vi "Periodic Tasks.vi"(8 "error in":errorcluster) -> ()   [LabVIEW 2016]
doc: "This VI runs in parallel to other tasks. It can contain as many user-defined periodic loops as you need. These can carry out PID or other sorts of timed response."
uses:
  <vilib>/Rock Robotics/WPI/Utilities/WPI_GetSetVariantRefNum.vi
  <vilib>/Rock Robotics/Network Tables/NT Write Number.vi
  2_11_17/Systems/Global 1.vi
  <vilib>/Analysis/NI_AALBase.lvlib
  <vilib>/Instr/_visa.llb/VISA Configure Serial Port (Instr).vi
  <vilib>/Analysis/3filter.llb/IIR Filter (DBL).vi
panel:
  out "PSI":dbl
  in  "off set":dbl=55.0 format="%#_13g"
  out "read buffer":string="B:3,X:197.00,Y:124.00"
  in  "Search_Params":string[](array[string])=["B", "X", "Y", "W1", "H1", "W2", "H2"]
  out "Last Complete Message":string="B:2,X:197.00,Y:124.00,W1:9,H1:24,W2:9,H2:23"
  out "length":i32=43
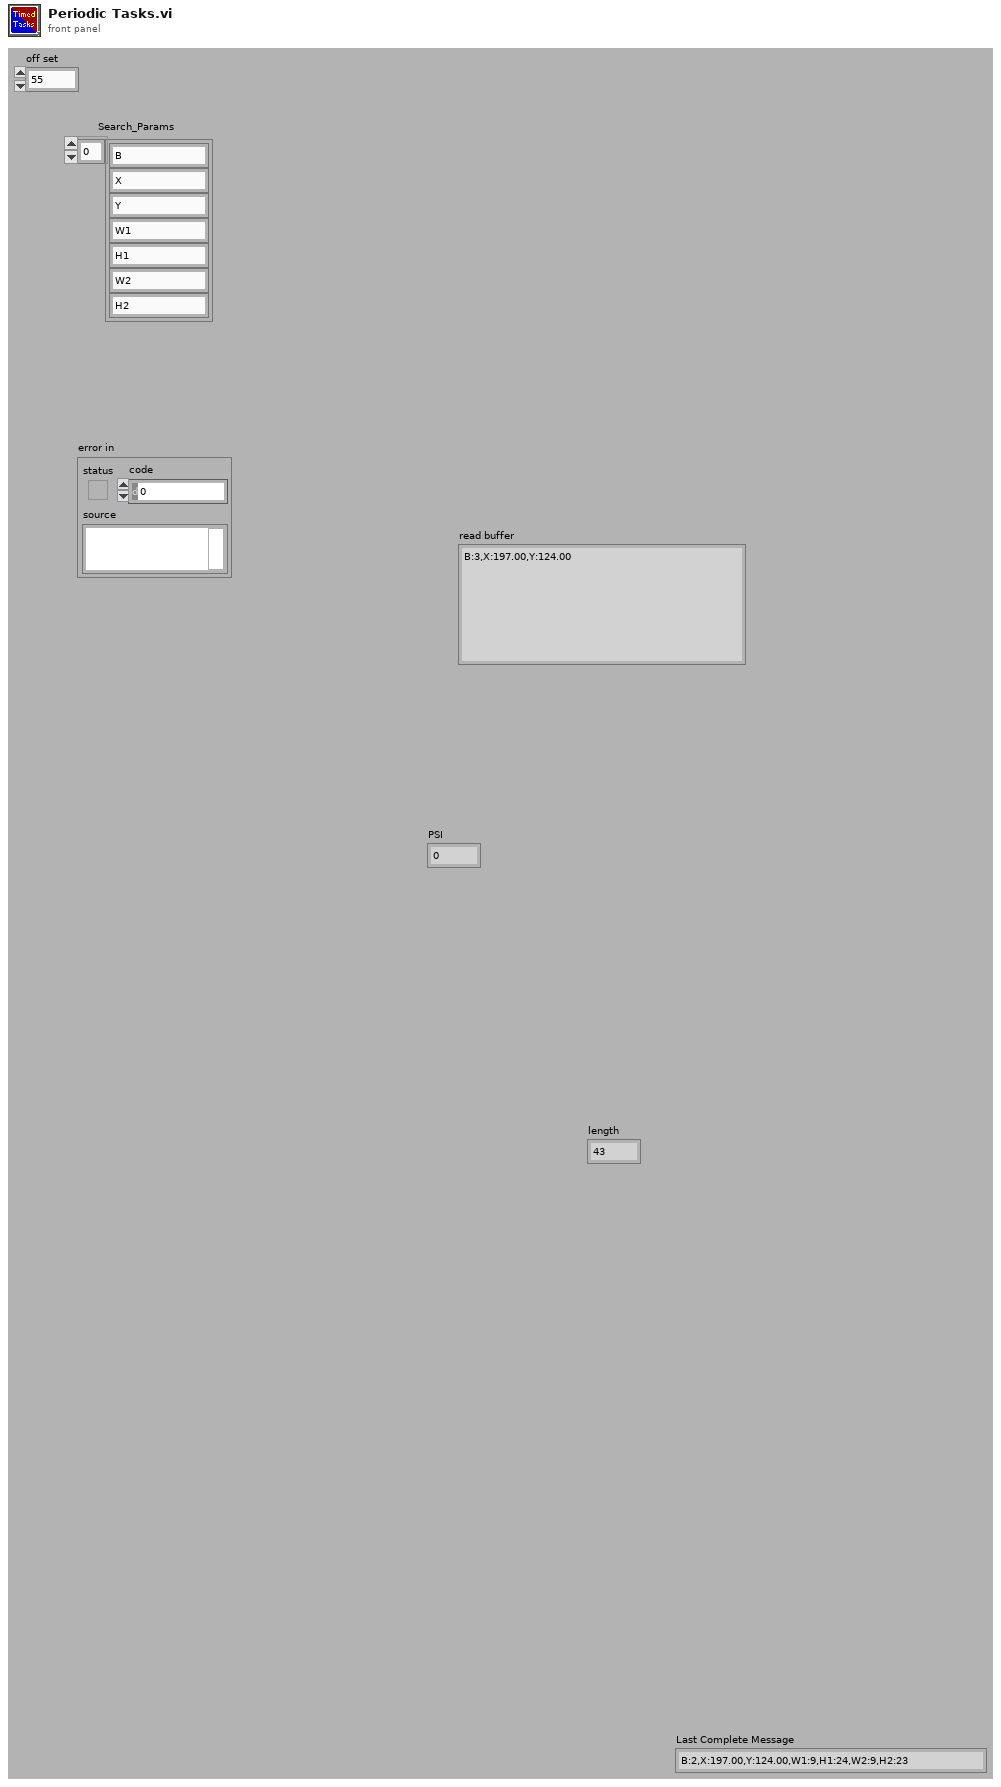
[diagram p1: front panel]
types:
  T1 = typedef "WPI_JoystickDevRef.ctl" = cluster{"Device":T2}
  T2 = typedef "WPI_JoystickDeviceEnum.ctl" = enum16{"USB 0", "USB 1", "USB 2", "USB 3", "USB 4", "USB 5"}
  T3 = typedef "WPI_AnalogChannelDevRef.ctl" = cluster{"DevStatus":errorcluster, "Analog Channel":T4}
  T4 = typedef "FPGA_AIChannel.ctl" = enum8{"AI 0", "AI 1", "AI 2", "AI 3", "AI MXP 0", "AI MXP 1", "AI MXP 2", "AI MXP 3", "Invalid"}
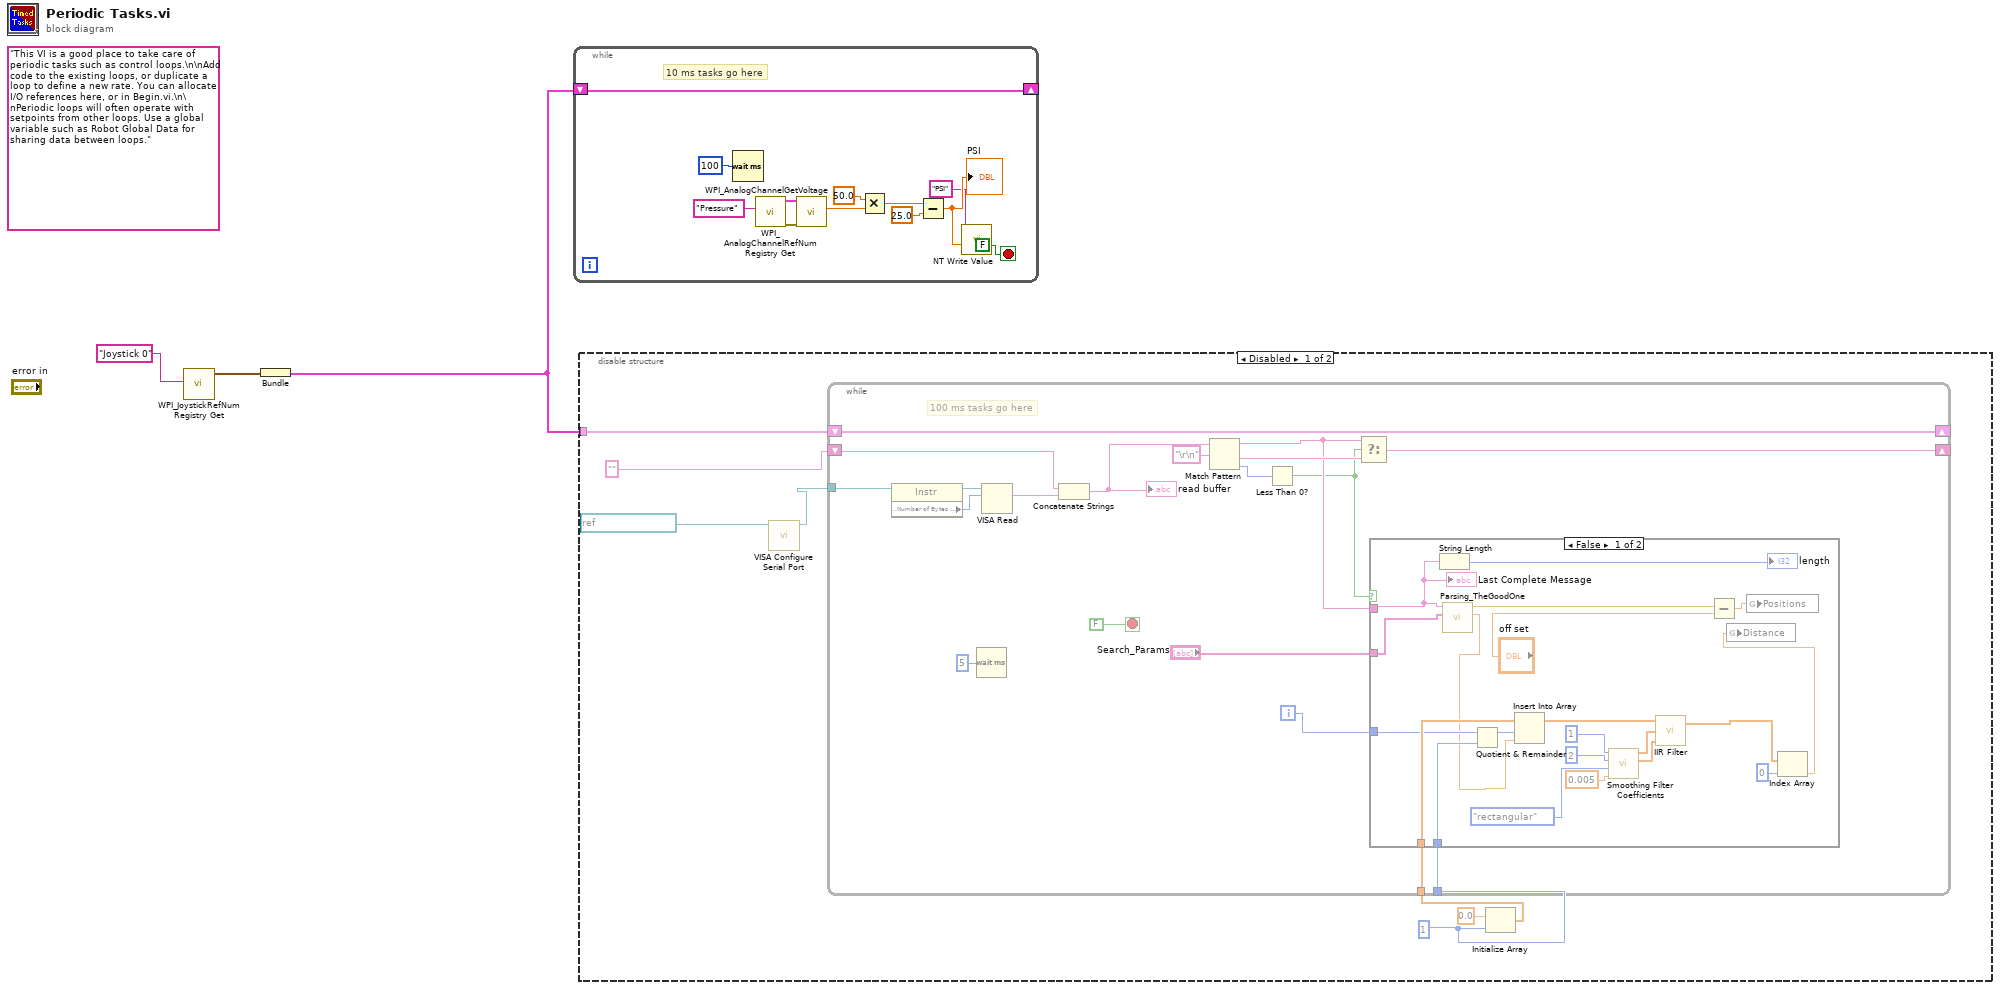
[diagram p0: block diagram]
diagram:
  (unwired) "This VI is a good place to take care of periodic tasks such as control loops.\n\nAdd code to the existing loops, or duplicate a loop to define a new rate. You can allocate I/O references here, or in Begin.vi.\n\nPeriodic loops will often operate with setpoints from other loops. Use a global variable such as Robot Global Data for sharing data between loops."
  n1 = call <vilib>:"WPI_JoystickRefNum Registry Get.vi"("refnum name"="Joystick 0") -> ("JoystickDevRef"=w2:T1)  [unwired: 1 in, 9 out]
  n2 = Bundle("JoystickDevRef"=w2) -> (w1:cluster{"JoystickDevRef":T1})  [unwired: 1 out]
  n3 = while {
    shift-right: [w13] -> _
    shift-left: w1 -> [w13]
    stop <- FALSE stop-if-true
    # "10 ms tasks go here"
    n4 = Wait (ms)(milliseconds to wait=u32 100) -> ()  [unwired: 1 out]
    n5 = call <vilib>:"WPI_AnalogChannelRefNum Registry Get.vi"("refnum name"="Pressure") -> ("error out"=w12:errorcluster, "AIDeviceRef"=w11:T3)  [unwired: 9 in]
    n6 = call <vilib>:"WPI_AnalogChannelGetVoltage.vi"("error in (no error)"=w12, "AIDeviceRef"=w11) -> ("Voltage"=w9:dbl)  [unwired: 7 in, 2 out]
    n7 = Multiply(x=50.0, y=w9) -> (x*y=w7:dbl)
    n8 = Subtract(x=w7, y=25.0) -> (x-y=w5:dbl)
    "PSI" <- w5
    n9 = call-poly <vilib>:"NT Write Value.vi"("Numeric"=w5, "Name"="PSI") -> ()  [unwired: 9 in, 1 out]
  }
  n10 = disable-structure shown="Disabled" {
    disable-tunnel: w1 -> [w19 _]
    frame Disabled {
      w22 = 1
      n11 = call-poly "VISA Configure Serial Port"("VISA resource name"=refnum<visa-resource-name> "ASRL2::INSTR") -> ("VISA resource name out"=w17:refnum<visa-resource-name>)  [unwired: 13 in, 1 out]
      n12 = Initialize Array(0.0 ("element"), w22) -> (w21:dbl[])
      n13 = while {
        shift-right: [w40] -> _
        shift-left: w19 -> [w40]
        tunnel: w17 -> [w35]
        shift-right: [w27] -> _
        shift-left: "" -> [w34]
        tunnel: w21 -> [w25]
        tunnel: w22 -> [w24]
        i -> [w23]
        stop <- FALSE stop-if-true
        # "100 ms tasks go here"
        n14 = property class="Instr"(reference=w35) -> (reference out=w39:refnum<visa-resource-name>, "Serial Settings:Number of Bytes at Serial Port"=w38:u32)  [unwired: 1 in, 1 out]
        n15 = Wait (ms)(milliseconds to wait=u32 5) -> ()  [unwired: 1 out]
        n16 = VISA Read(VISA resource name=w39, byte count=w38) -> (read buffer=w33:string)  [unwired: 1 in, 3 out]
        n17 = Concatenate Strings(w34, w33) -> (w32:string)
        "read buffer" <- w32
        n18 = Match Pattern(string=w32, regular expression="\r\n") -> (before substring=w28:string, after substring=w29:string, offset past match=w30:i32)  [unwired: 1 in, 1 out]
        n19 = Less Than 0?(x=w30) -> (x < 0?=w26:bool)
        n20 = Select(t=w28, s=w26, f=w29) -> (s? t:f=w27:string)
        n21 = case shown="False" w26 {
          tunnel: "Search_Params" -> [w61 _]
          tunnel: w28 -> [w60 _]
          tunnel: w25 -> [w48 _]
          tunnel: w24 -> [w47 _]
          tunnel: w23 -> [w46 _]
          frame False {
            n22 = String Length(string=w60) -> (length=→"length":i32)
            n23 = call "Parsing_TheGoodOne.vi"("Search_Params"=w61, "Input"=w60) -> ("Corrected distance"=w45:dbl, "Value-Reference"=w59:dbl)  [unwired: 6 in]
            n24 = Quotient & Remainder(x=w46, y=w47) -> (x-y*floor(x/y)=w49:i32)  [unwired: 1 out]
            n25 = Insert Into Array(array=w48, index=w49, new element=w45) -> (w50:dbl[])
            n26 = call <vilib>:"Smoothing Filter Coefficients.vi"("time constant"=0.005, "shape"=enum16{"rectangular", "triangular"}."rectangular", "half-width"=2, "type"=1) -> ("forward coefficients"=w52:dbl[], "reverse coefficients"=w53:dbl[])  [unwired: 5 in, 1 out]
            n27 = call-poly <vilib>:"IIR Filter.vi"("Forward Coefficients"=w52, "Reverse Coefficients"=w53, "X"=w50) -> ("Filtered X"=w44:dbl[])  [unwired: 1 in, 1 out]
            n28 = Subtract(x=w59, y="off set") -> (x-y=w57:dbl)
            n29 = global write "Global 1.vi" "Positions"(w57) -> ()
            n30 = Index Array(array=w44, index=0) -> (element=w42:dbl)
            n31 = global write "Global 1.vi" "Distance"(w42) -> ()
            "Last Complete Message" <- w60
          }
          frame True {
          }
        }
      }
    }
    frame Enabled {
    }
  }
